vi "New Preteleop.vi"() -> ()   [LabVIEW 2014]
uses:
  Pre-teleop States no tote.ctl
  Robot Global Data.vi
  Desired Arm Position.vi
  <vilib>/Rock Robotics/WPI/RobotDrive/WPI_RobotDriveGetSetRefNum.vi
panel:
  out "Enum":T1
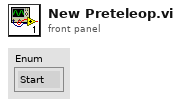
[diagram p1: front panel]
types:
  T1 = typedef "Pre-teleop States no tote.ctl" = enum16{"Start", "Grab Container", "Arms Up", "Turn towards loading station", "Drive towards loading station", "Stop"}
  T2 = typedef "WPI_RobotDriveDevRef.ctl" = cluster{"DevStatus":errorcluster, "Motors[]":T3[], "Square Inputs":bool, "Max Output":dbl}
  T3 = typedef "WPI_MotorControlDeviceRef.ctl" = cluster{"DeviceStatus":errorcluster, "Type":T4, "PWM":cluster{"Controller":T5, "PWM Channel":T6, "DeadBand":T7}, "CAN":cluster{"Device Number":u8, "Control Mode":T8, "Semaphore":T9, "Max Vout":dbl, "TalonSRX Control Mode":T10}, "Invert":bool, "TransformRef":T11, "InvTransformRef":T11}
  T4 = typedef "WPI_MotorControlType.ctl" = enum16{"PWM", "CAN", "CANTalonSRX"}
  T5 = typedef "FPGA_TypedefDigitalModule.ctl" = enum16{"Controller 1"}
  T6 = typedef "FPGA_DIOPWMChannel.ctl" = enum8{"PWM 0", "PWM 1", "PWM 2", "PWM 3", "PWM 4", "PWM 5", "PWM 6", "PWM 7", "PWM 8", "PWM 9", "PWM MXP 0", "PWM MXP 1", "PWM MXP 2", "PWM MXP 3", "PWM MXP 4", "PWM MXP 5", "PWM MXP 6", "PWM MXP 7", "PWM MXP 8", "PWM MXP 9", "Invalid"}
  T7 = typedef "WPI_PWMDeadband.ctl" = cluster{"Name":string, "maxPositivePwm":i32, "minPositivePwm":i32, "centerPwm":i32, "maxNegativePwm":i32, "minNegativePwm":i32, "angularRange":u16}
  T8 = typedef "WPI_CANJaguar_ControlMode.ctl" = enum8{"Percent VBus", "Current", "Speed", "Position", "Voltage"}
  T9 = typedef "Semaphore RefNum" = refnum<k1>
  T10 = typedef "WPI_CANTalonSRX_APIControlMode.ctl" = enum8{"Percent VBus", "Speed", "Position", "Slave", "Unchanged / Invalid"}
  T11 = typedef "WPI_PWMTransform_ConPane.ctl" = refnum<vi>
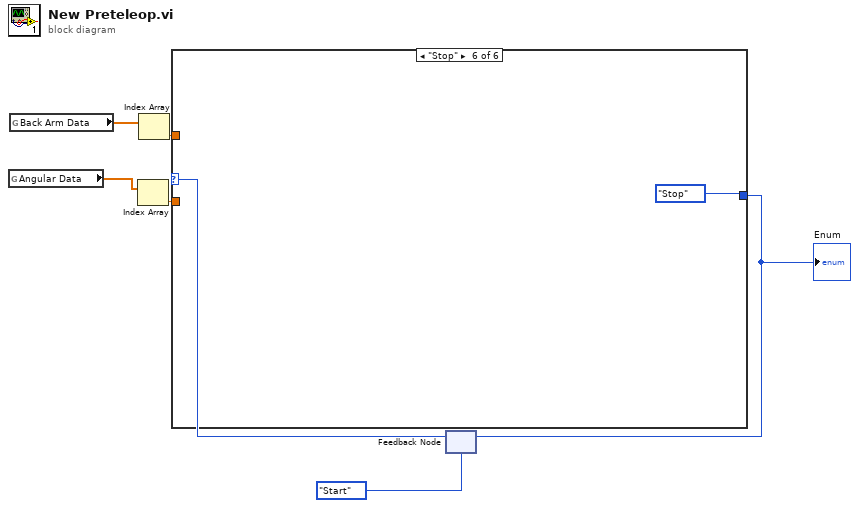
[diagram p0: block diagram]
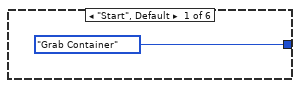
[diagram p2: hidden frame]
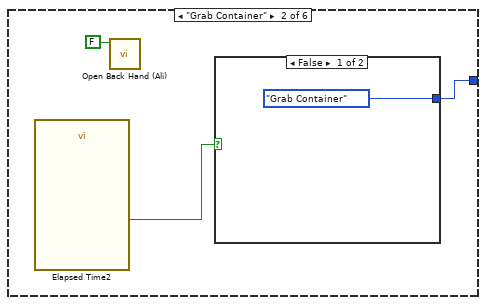
[diagram p3: hidden frame]
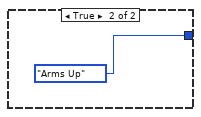
[diagram p4: hidden frame]
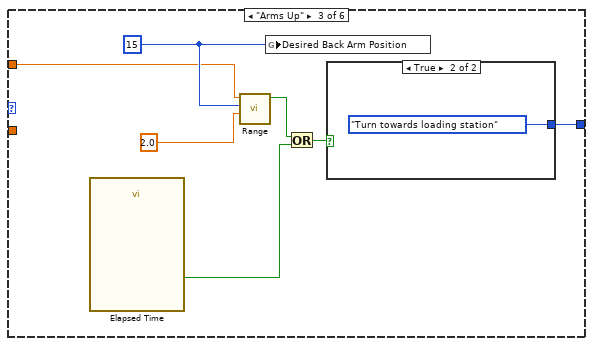
[diagram p5: hidden frame]
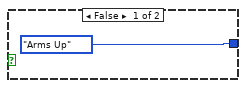
[diagram p6: hidden frame]
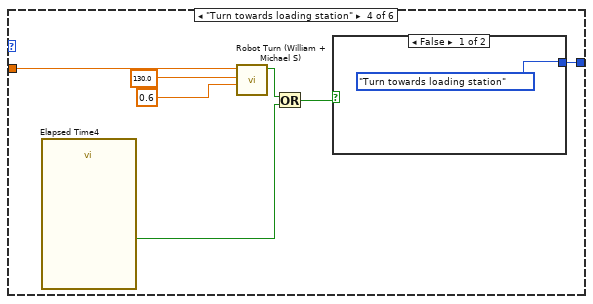
[diagram p7: hidden frame]
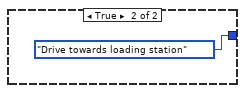
[diagram p8: hidden frame]
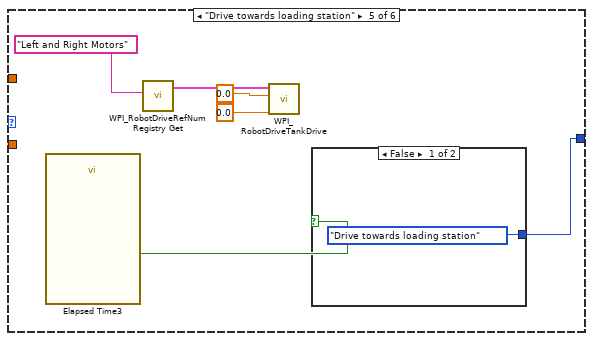
[diagram p9: hidden frame]
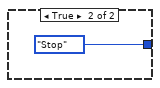
[diagram p10: hidden frame]
diagram:
  n1 = global read "Robot Global Data.vi" "Angular Data"() -> (w2:dbl[])
  n2 = global read "Robot Global Data.vi" "Back Arm Data"() -> (w4:dbl[])
  n3 = Index Array(array=w2) -> (element=w1:dbl)  [unwired: 1 in]
  n4 = Index Array(array=w4) -> (element=w3:dbl)  [unwired: 1 in]
  n5 = feedback #1(Pre-teleop_States_no_tote."Start") -> (w6:T1)
  n6 = case shown="\"Stop\"" w6 {
    tunnel: [Pre-teleop_States_no_tote."Grab Container" w9 w17 w26 w32 Pre-teleop_States_no_tote."Stop"] -> w5
    tunnel: w3 -> [_ _ w19 _ _ _]
    tunnel: w1 -> [_ _ _ w29 _ _]
    frame "Start", Default {
    }
    frame "Grab Container" {
      n7 = call "Elapsed Time2"() -> ("Time has Elapsed"=w10:bool)  [unwired: 12 in, 7 out]
      n8 = call "Open Back Hand (Ali).vi"("Open?"=FALSE) -> ()  [unwired: 11 in]
      n9 = case shown="False" w10 {
        tunnel: [Pre-teleop_States_no_tote."Grab Container" Pre-teleop_States_no_tote."Arms Up"] -> w9
        frame False {
        }
        frame True {
        }
      }
    }
    frame "Arms Up" {
      w20 = 15
      n10 = call "Elapsed Time"() -> ("Time has Elapsed"=w14:bool)  [unwired: 12 in, 7 out]
      n11 = call "Range.vi"("Range"=2.0, "Input"=w20, "In Range of"=w19) -> ("In Range?"=w15:bool)  [unwired: 8 in]
      n12 = global write "Desired Arm Position.vi" "Desired Back Arm Position"(w20) -> ()
      n13 = Or(x=w15, y=w14) -> (x .or. y?=w16:bool)
      n14 = case shown="True" w16 {
        tunnel: [Pre-teleop_States_no_tote."Arms Up" Pre-teleop_States_no_tote."Turn towards loading station"] -> w17
        frame False {
        }
        frame True {
        }
      }
    }
    frame "Turn towards loading station" {
      n15 = call "Elapsed Time4"() -> ("Time has Elapsed"=w24:bool)  [unwired: 12 in, 7 out]
      n16 = call "Robot Turn (William + Michael S).vi"("X axis value"=0.6, "Desired Degree"=130.0, "Gyro Degrees"=w29) -> ("Stop"=w25:bool)  [unwired: 8 in]
      n17 = Or(x=w25, y=w24) -> (x .or. y?=w23:bool)
      n18 = case shown="False" w23 {
        tunnel: [Pre-teleop_States_no_tote."Turn towards loading station" Pre-teleop_States_no_tote."Drive towards loading station"] -> w26
        frame False {
        }
        frame True {
        }
      }
    }
    frame "Drive towards loading station" {
      n19 = call "Elapsed Time3"() -> ("Time has Elapsed"=w33:bool)  [unwired: 12 in, 7 out]
      n20 = call <vilib>:"WPI_RobotDriveRefNum Registry Get.vi"("refnum name"="Left and Right Motors") -> ("RobotDriveDevRef"=w37:T2)  [unwired: 9 in, 1 out]
      n21 = call <vilib>:"WPI_RobotDriveTankDrive.vi"("Right axis value"=0.0, "Left axis value"=0.0, "RobotDriveDevRef"=w37) -> ()  [unwired: 6 in, 3 out]
      n22 = case shown="False" w33 {
        tunnel: [Pre-teleop_States_no_tote."Drive towards loading station" Pre-teleop_States_no_tote."Stop"] -> w32
        frame False {
        }
        frame True {
        }
      }
    }
    frame "Stop" {
    }
  }
  "Enum" <- w5
  n23 = feedback-in #1(w5) -> ()
